vi "extractcolor.vi"(8 "error in (no error)":errorcluster, 10 "Color Mode":u16(ring) items=["RGB", "HSL", "HSV", "HSI"], 11 "Image Src":T1) -> (0 "error out Extract":errorcluster, 1 "Blue or Luma or Val or Inten Plane out":T1, 2 "Green or Sat Plane out":T1, 3 "Red or Hue Plane out":T1)   [LabVIEW 2017]
uses:
  <vilib>/vision/Image Controls.llb/IMAQ Image.ctl
  <vilib>/vision/NI_Vision_Development_Module.lvlib
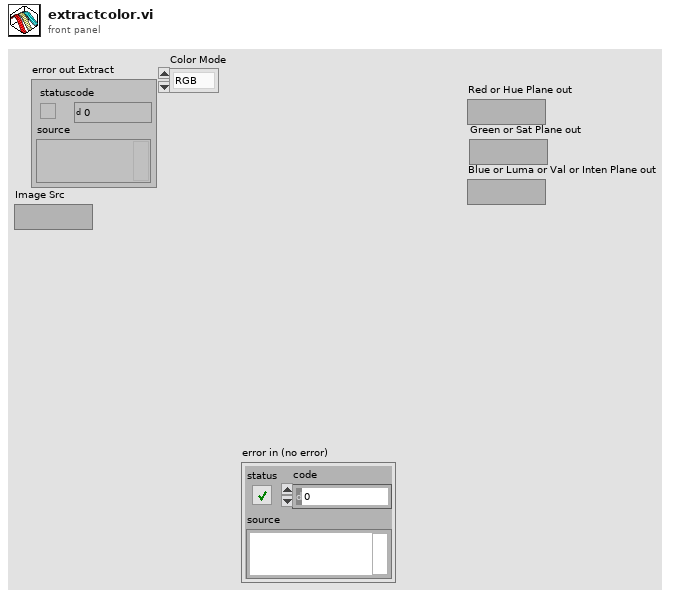
[diagram p1: front panel]
types:
  T1 = typedef "IMAQ Image.ctl" = refnum<image>
  T2 = typedef "Image Type" = u32
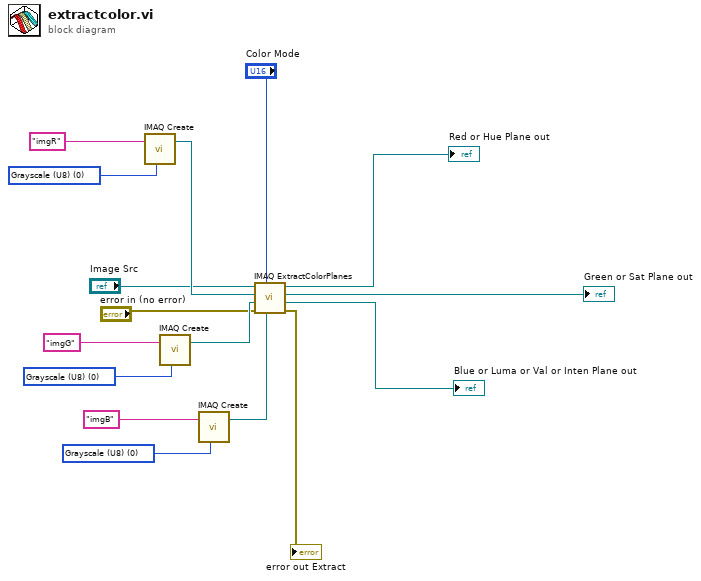
[diagram p0: block diagram]
diagram:
  w7 = T2 0 items=["Grayscale (U8)", "Grayscale (I16)", "Grayscale (SGL)", "Complex (CSG)", "RGB (U32)", "HSL (U32)", "RGB (U64)", "Grayscale (U16)"] ("Image Type")
  w10 = T2 0 items=["Grayscale (U8)", "Grayscale (I16)", "Grayscale (SGL)", "Complex (CSG)", "RGB (U32)", "HSL (U32)", "RGB (U64)", "Grayscale (U16)"] ("Image Type")
  w14 = T2 0 items=["Grayscale (U8)", "Grayscale (I16)", "Grayscale (SGL)", "Complex (CSG)", "RGB (U32)", "HSL (U32)", "RGB (U64)", "Grayscale (U16)"] ("Image Type")
  n1 = call "IMAQ Create"("Image Name"="imgR", "Image Type"=w14) -> ("New Image"=w13:T1)  [unwired: 3 in, 1 out]
  n2 = call "IMAQ Create"("Image Name"="imgG", "Image Type"=w10) -> ("New Image"=w9:T1)  [unwired: 3 in, 1 out]
  n3 = call "IMAQ Create"("Image Name"="imgB", "Image Type"=w7) -> ("New Image"=w6:T1)  [unwired: 3 in, 1 out]
  n4 = call "IMAQ ExtractColorPlanes"("Blue or Luma or Val or Inten Plane"=w6, "Color Mode"="Color Mode", "error in (no error)"="error in (no error)", "Green or Sat Plane"=w9, "Red or Hue Plane"=w13, "Image Src"="Image Src") -> ("error out"=→"error out Extract":errorcluster, "Blue or Luma or Val or Inten Plane out"=→"Blue or Luma or Val or Inten Plane out":T1, "Green or Sat Plane out"=→"Green or Sat Plane out":T1, "Red or Hue Plane out"=→"Red or Hue Plane out":T1)  [unwired: 2 in]
